vi "Start measurements.vi"(6 "Syncronize measurements":bool=TRUE, 8 "error in (no error)":errorcluster, 9 "Repeat times":i32=-1, 10 "Measurements":string[](array[string]), 11 "Common Measurements in":refnum<class "Common Measurements.lvclass">) -> (0 "error out":errorcluster, 3 "Common Measurements out":refnum<class "Common Measurements.lvclass">)   [LabVIEW 2015, in "Common Measurements.lvclass"]
uses:
  Common Measurements.lvclass
  Common Measurements.lvclass/Common Measurements.ctl
  Mag Lab Measure Base/Mag Lab Measure Base.lvclass/Mag Lab Measure Base.ctl
  Common Measurements Interface Messages/Write File Path Msg/Write File Path Msg.lvclass/Write File Path Msg.ctl
  <vilib>/ActorFramework/Message Enqueuer/Message Enqueuer.lvclass/Message Enqueuer.ctl
  Common Measurements Interface Messages/Set Running Msg/Set Running Msg.lvclass/Set Running Msg.ctl
  MagLabGraph Messages/Add file Msg/Add file Msg.lvclass/Add file Msg.ctl
  <vilib>/ActorFramework/Message Enqueuer/Enqueue.vi
  <vilib>/ActorFramework/Message Priority Queue/Priority Enqueue.vi
  <vilib>/ActorFramework/Message Enqueuer/Message Enqueuer.lvclass
  Common Measurements Interface Messages/Write File Path Msg/Write File Path Msg.lvclass
  Common Measurements Interface Messages/Set Running Msg/Set Running Msg.lvclass
  MagLabGraph Messages/Add file Msg/Add file Msg.lvclass
  Mag Lab Measure Controller/Mag Lab Measure Controller.lvclass
  Mag Lab Measure Base/Mag Lab Measure Base.lvclass
  Mag Lab Error Handler/Mag Lab Error Handler.lvclass
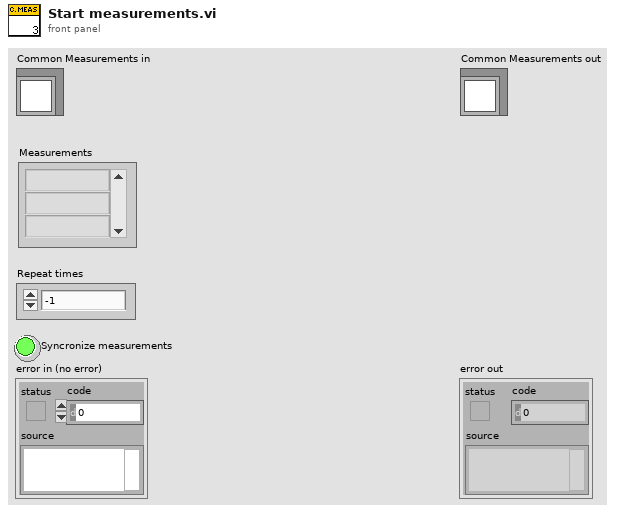
[diagram p1: front panel]
types:
  T1 = enum16{"open", "open or create", "create or replace", "create", "open (read-only)"}
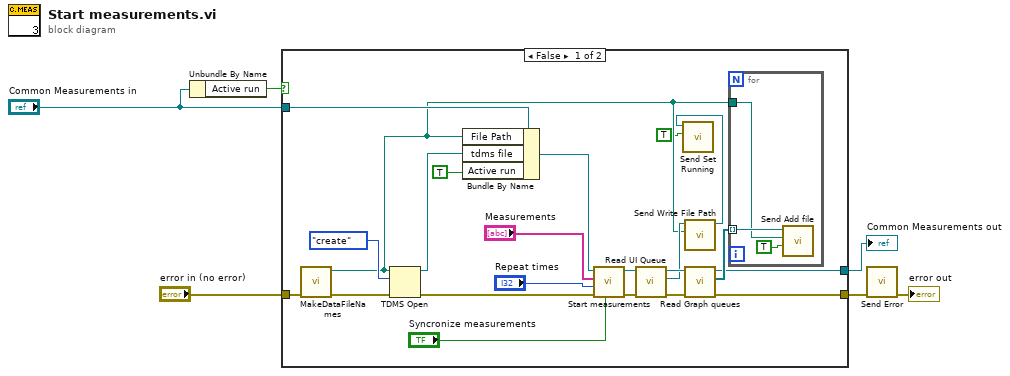
[diagram p0: block diagram]
diagram:
  n1 = Unbundle By Name("Common Measurements in") -> ("Active run"=w4:bool)
  n2 = case shown="False" w4 {
    tunnel: [w14 w33] -> w2
    tunnel: "error in (no error)" -> [w25 w33]
    tunnel: "Common Measurements in" -> [w19 w32]
    tunnel: [w13 w32] -> w3
    frame False {
      n3 = call "MakeDataFileNames.vi"("Error In"=w25) -> ("Error Out"=w27:errorcluster, "Data File  Path"=w15:path)  [unwired: 7 in, 2 out]
      n4 = TDMS Open(8:w27, 10:T1."create" ("operation (0:open)"), 11:w15) -> (0:w10:errorcluster, 3:w18:refnum<k34>)  [unwired: 4 in]
      n5 = Bundle By Name(cluster=w19, "File Path"=w15, "tdms file"=w18, "Active run"=TRUE) -> (w11:refnum<class "Common Measurements.lvclass">)
      n6 = call-parent "Start measurements.vi"("Syncronize measurements"="Syncronize measurements", "error in (no error)"=w10, "Repeat times"="Repeat times", "Measurements"="Measurements", "Mag Lab Measure Controller in"=w11) -> ("error out"=w24:errorcluster, "Mag Lab Measure Controller out"=w23:refnum<class "Common Measurements.lvclass">)  [unwired: 5 in]
      n7 = call "Read UI Queue.vi"("error in (no error)"=w24, "Mag Lab Measure Base in"=w23) -> ("error out"=w21:errorcluster, "Actor Framework.lvlib:Message Enqueuer"=w16:refnum<class "Message Enqueuer.lvclass">, "Mag Lab Measure Base out"=w22:refnum<class "Common Measurements.lvclass">)  [unwired: 7 in]
      n8 = call "Send Write File Path.vi"("File Path"=w15, "Message Enqueuer"=w16) -> ("Message Enqueuer out"=w7:refnum<class "Message Enqueuer.lvclass">)  [unwired: 8 in, 1 out]
      n9 = call "Send Set Running.vi"("Running"=TRUE, "Message Enqueuer"=w7) -> ()  [unwired: 8 in, 2 out]
      n10 = call "Read Graph queues.vi"("error in (no error)"=w21, "Mag Lab Measure Base in"=w22) -> ("error out"=w14:errorcluster, "Graph queues"=w20:refnum<class "Message Enqueuer.lvclass">[], "Mag Lab Measure Base out"=w13:refnum<class "Common Measurements.lvclass">)  [unwired: 7 in]
      n11 = for {
        tunnel: w20 -> [w31] mode=indexing
        tunnel: w15 -> [w30]
        n12 = call "Send Add file.vi"("Insert in front"=TRUE, "File Path Control"=w30, "Message Enqueuer"=w31) -> ()  [unwired: 7 in, 2 out]
      }
    }
    frame True {
    }
  }
  "Common Measurements out" <- w3
  n13 = call "Send Error.vi"("error in (no error)"=w2) -> ("error out"=→"error out":errorcluster)  [unwired: 9 in, 1 out]
